vi "RemoveUsedSeriesJSONs.vi"() -> ()   [LabVIEW 2024]
uses:
  Marvel_API/TypeDefs/series--cluster.ctl
  <vilib>/addons/_JKI.lib/Serialization/JSON/JKI JSON Serialization.lvlib
panel:
  out "deleted":bool
  in  "series data path":path=path "D:/data/series"
  out "current series path":path
  out "current comic path":path
  in  "repo path":path=path "D:/Comics/Marvel"
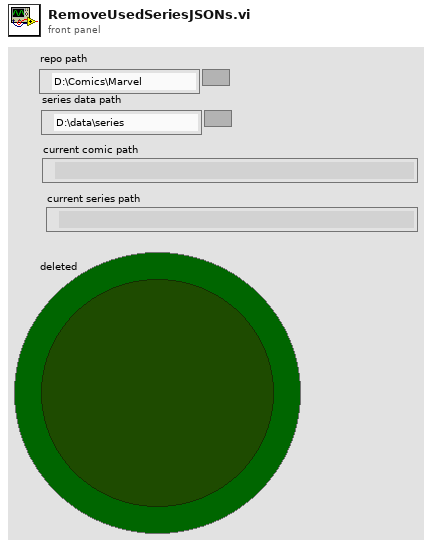
[diagram p1: front panel]
types:
  T1 = typedef "series--cluster.ctl" = cluster{"id":i32, "title":string, "description":string, "resourceURI":string, "urls":cluster{"type":string, "url":string}[], "startYear":i32, "endYear":i32, "rating":string, "type":string, "modified":variant, "thumbnail":cluster{"path":string, "extension":string}, "creators":cluster{"available":i32, "returned":i32, "collectionURI":string, "items":cluster{"resourceURI":string, "name":string, "role":string}[]}, "comics":cluster{"available":i32, "returned":i32, "collectionURI":string, "items":cluster{"resourceURI":string, "name":string}[]}, "characters":cluster{"available":i32, "returned":i32, "collectionURI":string, "items":cluster{"resourceURI":string, "name":string}[]}, "stories":cluster{"available":i32, "returned":i32, "collectionURI":string, "items":cluster{"resourceURI":string, "name":string, "type":string}[]}, "events":cluster{"available":i32, "returned":i32, "collectionURI":string, "items":cluster{"resourceURI":string, "name":string}[]}, "next":variant, "previous":variant}
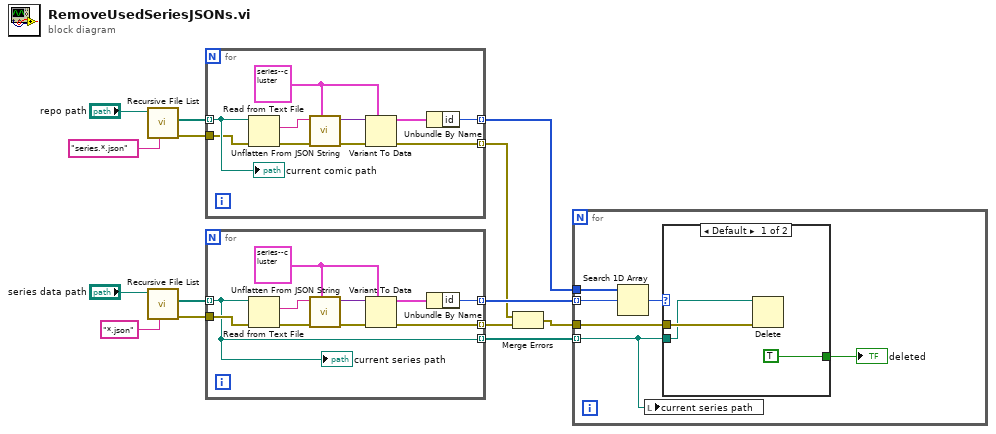
[diagram p0: block diagram]
diagram:
  n1 = call <vilib>:"Recursive File List.vi"("pattern"="series.*.json", "Folder Path"="repo path") -> ("error out"=w11:errorcluster, "All Files in Dir"=w13:path[])  [unwired: 5 in, 3 out]
  n2 = call <vilib>:"Recursive File List.vi"("pattern"="*.json", "Folder Path"="series data path") -> ("error out"=w10:errorcluster, "All Files in Dir"=w8:path[])  [unwired: 5 in, 3 out]
  n3 = for {
    tunnel: w13 -> [w24] mode=indexing
    tunnel: w11 -> [w23]
    tunnel: [w16] -> w4 mode=indexing
    tunnel: [w15] -> w2 mode=indexing
    w18 = T1 {"id"=0, "title"="", "description"="", "resourceURI"="", "urls"=[], "startYear"=0, "endYear"=0, "rating"="", "type"="", "modified"=variant, "thumbnail"={"path"="", "extension"=""}, "creators"={"available"=0, "returned"=0, "collectionURI"="", "items"=[]}, "comics"={"available"=0, "returned"=0, "collectionURI"="", "items"=[]}, "characters"={"available"=0, "returned"=0, "collectionURI"="", "items"=[]}, "stories"={"available"=0, "returned"=0, "collectionURI"="", "items"=[]}, "events"={"available"=0, "returned"=0, "collectionURI"="", "items"=[]}, "next"=variant, "previous"=variant} ("Cluster")
    n4 = Read from Text File(file (use dialog)=w24, error in=w23) -> (text=w22:string, error out=w21:errorcluster)  [unwired: 2 in, 2 out]
    n5 = call <vilib>:"Unflatten From JSON String.vi"("Type and Defaults"=w18, "error in (no error)"=w21, "JSON String"=w22) -> ("error out"=w20:errorcluster, "Variant"=w19:variant)  [unwired: 7 in]
    n6 = Variant To Data(error in=w20, type=w18, Variant=w19) -> (data=w17:T1, error out=w15:errorcluster)
    n7 = Unbundle By Name(w17) -> ("id"=w16:i32)
    "current comic path" <- w24
  }
  n8 = for {
    tunnel: w8 -> [w26] mode=indexing
    tunnel: w10 -> [w34]
    tunnel: [w27] -> w5 mode=indexing
    tunnel: [w26] -> w6 mode=indexing
    tunnel: [w25] -> w3 mode=indexing
    w29 = T1 {"id"=0, "title"="", "description"="", "resourceURI"="", "urls"=[], "startYear"=0, "endYear"=0, "rating"="", "type"="", "modified"=variant, "thumbnail"={"path"="", "extension"=""}, "creators"={"available"=0, "returned"=0, "collectionURI"="", "items"=[]}, "comics"={"available"=0, "returned"=0, "collectionURI"="", "items"=[]}, "characters"={"available"=0, "returned"=0, "collectionURI"="", "items"=[]}, "stories"={"available"=0, "returned"=0, "collectionURI"="", "items"=[]}, "events"={"available"=0, "returned"=0, "collectionURI"="", "items"=[]}, "next"=variant, "previous"=variant} ("Cluster")
    n9 = Read from Text File(file (use dialog)=w26, error in=w34) -> (text=w33:string, error out=w32:errorcluster)  [unwired: 2 in, 2 out]
    n10 = call <vilib>:"Unflatten From JSON String.vi"("Type and Defaults"=w29, "error in (no error)"=w32, "JSON String"=w33) -> ("error out"=w31:errorcluster, "Variant"=w30:variant)  [unwired: 7 in]
    n11 = Variant To Data(error in=w31, type=w29, Variant=w30) -> (data=w28:T1, error out=w25:errorcluster)
    n12 = Unbundle By Name(w28) -> ("id"=w27:i32)
    "current series path" <- w26
  }
  n13 = Merge Errors(w2, w3) -> (w1:errorcluster)
  n14 = for {
    tunnel: w6 -> [w37] mode=indexing
    tunnel: w5 -> [w39] mode=indexing
    tunnel: w4 -> [w40]
    tunnel: w1 -> [w36]
    n15 = Search 1D Array(1D array=w40, element=w39) -> (index of element=w38:i32)  [unwired: 1 in]
    n16 = local write "current series path"(w37) -> ()
    n17 = case shown="Default" w38 {
      tunnel: w37 -> [w42 _]
      tunnel: w36 -> [w43 _]
      tunnel: [TRUE _] -> w35
      frame Default {
        n18 = Delete(path (use dialog)=w42, error in=w43) -> ()  [unwired: 3 in, 3 out]
      }
      frame -1 {
      }
    }
    "deleted" <- w35
  }
